vi "Left Click.vi"(4 "Top  VI":refnum<vi>, 6 "Coords":T2, 7 "object refs":T1, 8 "error in (no error)":errorcluster, 9 "line name":string, 10 "Table Manager in":refnum<class "Table Manager.lvclass">, 11 "Tag Channel Column in":refnum<class "Mapping Column.lvclass">) -> (0 "error out":errorcluster, 1 "Discard":bool, 2 "Table Manager out":refnum<class "Table Manager.lvclass">, 3 "Tag Channel Column out":refnum<class "Mapping Column.lvclass">)   [LabVIEW 2013, in "Table Manager.lvlib" / "Mapping Column.lvclass"]
uses:
  Mapping Column.lvclass
  <vilib>/Utility/miscctls.llb/LVPoint32TypeDef.ctl
  Table Manager/object ref.ctl
  <vilib>/NI/DCAF/Tag Editor Core/Configuration Editor/Classes/Engine Parent/Engine Parent Editor Node.lvclass
  <vilib>/NI/DCAF/Tag Editor Core/Configuration Editor/Classes/Module editor node/module editor node.lvclass
  Table Manager/Table Manager.lvclass
  Table Manager/Table Manager.lvclass/Table Manager.ctl
  Mapping Column.lvclass/Mapping Column.ctl
  <vilib>/NI/Tag Bus Module Framework/module configuration/TBM module configuration.lvclass
  <vilib>/NI/Tag Bus/tag/tag descriptor.lvclass/tag descriptor.ctl
  Table Manager/Read ATM.vi
  <vilib>/NI/Tag Bus/tag/read tag name.vi
  <vilib>/NI/DCAF/Tag Editor Core/Configuration Editor/Classes/Module editor node/Read Module Configuration.vi
  <vilib>/NI/Tag Bus Module Framework/channel/TBM channel.lvclass
  <vilib>/NI/Tag Bus/tag/tag descriptor.lvclass
  Table Manager.lvlib
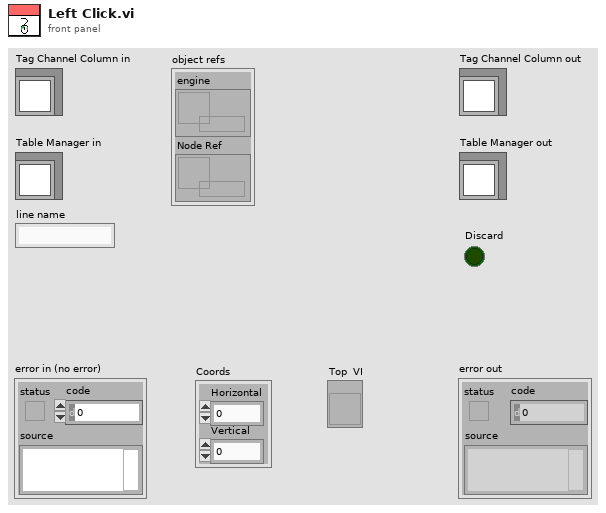
[diagram p1: front panel]
types:
  T1 = typedef "Table Manager.lvlib/Table Manager.lvclass/object ref.ctl" = cluster{"engine":refnum<data-value>, "Node Ref":refnum<data-value>}
  T2 = typedef "LVPoint32TypeDef.ctl" = cluster{"Horizontal":i32, "Vertical":i32}
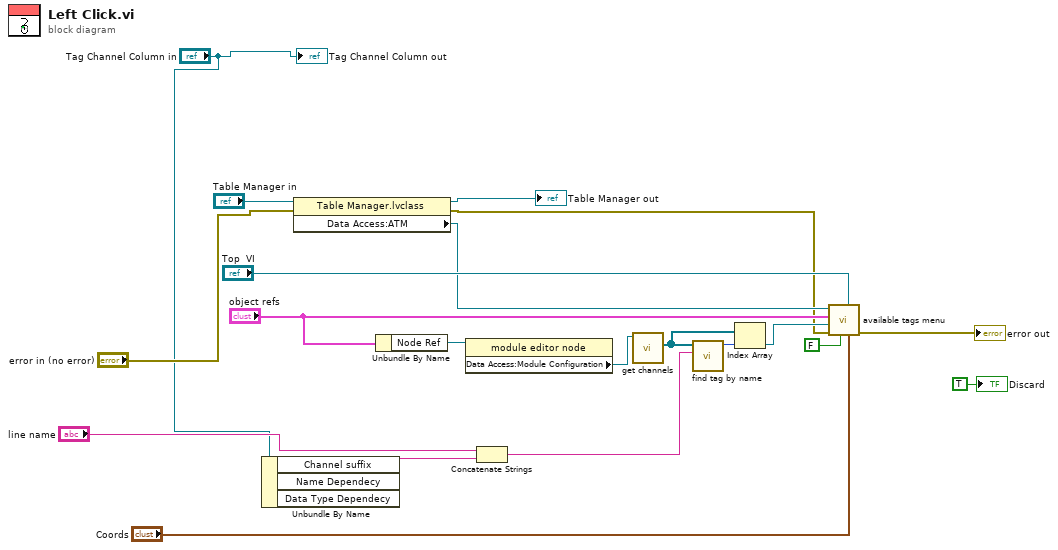
[diagram p0: block diagram]
diagram:
  n1 = Unbundle By Name("Tag Channel Column in") -> ("Channel suffix"=w9:string)  [unwired: 2 out]
  n2 = property class="Table Manager.lvclass"(reference="Table Manager in", error in="error in (no error)") -> (reference out=→"Table Manager out":refnum<class "Table Manager.lvclass">, error out=w5:errorcluster, "Data Access:ATM"=w12:refnum<user-event>)
  n3 = Unbundle By Name("object refs") -> ("Node Ref"=w16:refnum<data-value>)
  n4 = property class="module editor node"(reference=w16) -> ("Data Access:Module Configuration"=w17:refnum<class "TBM module configuration.lvclass">)  [unwired: 1 in, 2 out]
  n5 = Concatenate Strings("line name", w9) -> (w7:string)
  n6 = call-dynamic "get channels.vi"("module configuration in"=w17) -> ("channels"=w18:refnum<class "TBM channel.lvclass">[])  [unwired: 9 in, 1 out]
  n7 = call <vilib>:"find tag by name.vi"("name"=w7, "tags in"=w18) -> ("index"=w20:i32)  [unwired: 9 in]
  n8 = Index Array(array=w18, index=w20) -> (element=w19:refnum<class "TBM channel.lvclass">)
  n9 = call "available tags menu.vi"("Point32"="Coords", "parent vi reference"="Top  VI", "Screen"=FALSE, "error in"=w5, "channel to map to"=w19, "object ref"="object refs", "ATM"=w12) -> ("error out"=→"error out":errorcluster)  [unwired: 4 in]
  "Tag Channel Column out" <- "Tag Channel Column in"
  "Discard" <- TRUE ("Discard")
